vi "S2C_VAR_MenuProcess.vi"(8 "Error In":errorcluster, 10 "ItemTag":string, 11 "CtrlRef":refnum<vi>) -> (0 "Error Out":errorcluster)   [LabVIEW 2015]
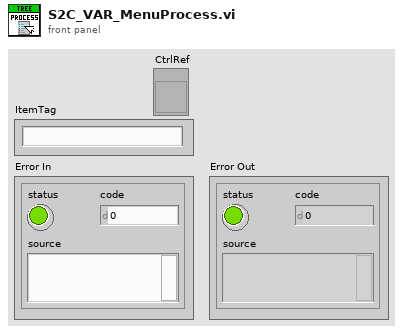
[diagram p1: front panel]
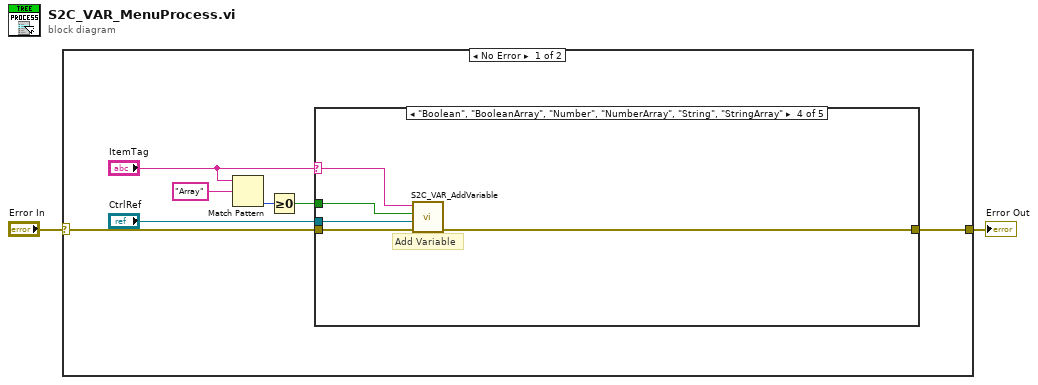
[diagram p0: block diagram]
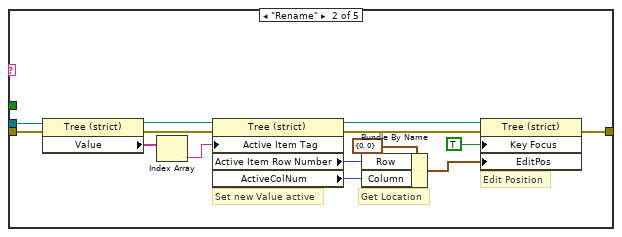
[diagram p3: hidden frame]
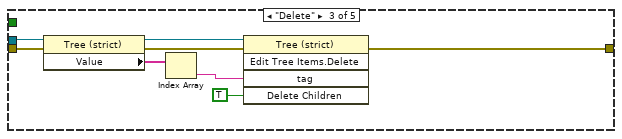
[diagram p4: hidden frame]
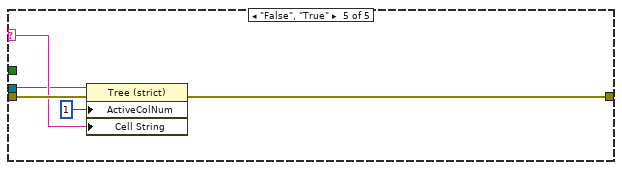
[diagram p5: hidden frame]
diagram:
  n1 = case shown="No Error" "Error In" {
    selector: "Error In" -> [w6 w43]
    tunnel: [w4 w43] -> w1
    frame No Error {
      n2 = Match Pattern(string="ItemTag", regular expression="Array" ("string")) -> (offset past match=w8:i32)  [unwired: 1 in, 3 out]
      n3 = Greater Or Equal To 0?(x=w8) -> (x >= 0?=w7:bool)
      n4 = case shown="\"Boolean\", \"BooleanArray\", \"Number\", \"NumberArray\", \"String\", \"StringArray\"" "ItemTag" {
        selector: "ItemTag" -> [_ _ _ w34 w39]
        tunnel: [w10 w18 w32 w37 w41] -> w4
        tunnel: w6 -> [w10 w16 w31 w36 w42]
        tunnel: w7 -> [_ _ _ w35 _]
        tunnel: "CtrlRef" -> [_ w15 w25 w33 w38]
        frame "Other", Default {
        }
        frame "Rename" {
          # "Edit Position"
          # "Get Location"
          # "Set new Value active"
          n5 = property class="Tree (strict)"(reference=w15, error in=w16) -> (reference out=w12:refnum<vi>, error out=w11:errorcluster, "Value"=w14:string[])
          n6 = Index Array(array=w14) -> (element=w13:string)  [unwired: 1 in]
          n7 = property class="Tree (strict)"(reference=w12, error in=w11, "Active Item Tag"=w13) -> (reference out=w23:refnum<vi>, error out=w24:errorcluster, "Active Item Row Number"=w21:i32, "ActiveColNum"=w17:i32)
          n8 = Bundle By Name(cluster=cluster{"Row":i32, "Column":i32} {"Row"=0, "Column"=0} ("Edit Position"), "Row"=w21, "Column"=w17) -> (w20:cluster{"Row":i32, "Column":i32})
          n9 = property class="Tree (strict)"(reference=w23, error in=w24, "Key Focus"=TRUE, "EditPos"=w20) -> (error out=w18:errorcluster)  [unwired: 1 out]
        }
        frame "Delete" {
          n10 = property on="Property Node" class="Tree (strict)"(reference=w25, error in=w31) -> (reference out=w26:refnum<vi>, error out=w30:errorcluster, "Value"=w29:string[])
          n11 = Index Array(array=w29) -> (element=w28:string)  [unwired: 1 in]
          n12 = invoke on="Invoke Node" class="Tree (strict)" method="Edit Tree Items.Delete"(reference=w26, error in=w30, "tag"=w28, "Delete Children"=TRUE ("Delete Children?")) -> (error out=w32:errorcluster)  [unwired: 1 in, 4 out]
        }
        frame "Boolean", "BooleanArray", "Number", "NumberArray", "String", "StringArray" {
          # "Add Variable"
          n13 = call "S2C_VAR_AddVariable.vi"("Error In"=w36, "TreeRef"=w33, "Array?"=w35, "Type"=w34) -> ("Error Out"=w37:errorcluster)  [unwired: 7 in]
        }
        frame "False", "True" {
          n14 = property on="Property Node" class="Tree (strict)"(reference=w38, error in=w42, "ActiveColNum"=1 ("Active Cell:Active Column Number"), "Cell String"=w39) -> (error out=w41:errorcluster)  [unwired: 1 out]
        }
      }
    }
    frame Error {
    }
  }
  "Error Out" <- w1
